vi "Micro-PL Drive Calibration v10.0.0.vi"() -> ()   [LabVIEW 2010]
uses:
  <vilib>/Utility/miscctls.llb/LVPointTypeDef.ctl
  subvi/ESA-C/TypeDefs/ESA-C Connection Settings.ctl
  <vilib>/Utility/file.llb/Write To Spreadsheet File (DBL).vi
panel:
  in  "GPIB-Port":u8=4 max=150 step=1
  in  "Start":bool
  out "Voltages":ext[][](array[numeric])
  out "Current Voltage":ext caption="Current (V)" format="%.1f"
  in  "Axis":u16(ring)=1 items=["X"=1, "Y"=2, "Z"=3]
  out "Progress":u8(slide) max=10 scale=0.0..100.0
  in  "Exit":bool
  in  "Voltage Step":dbl=1.0 caption="Step (V)" min=0.1 max=30.0 step=0.1
  # "Drive Calibration"
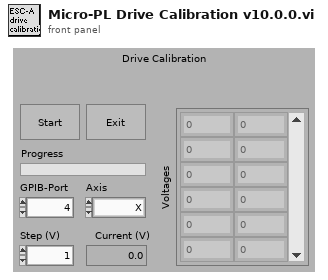
[diagram p1: front panel]
types:
  T1 = typedef "LVPointTypeDef.ctl" = cluster{"Horizontal":i16, "Vertical":i16}
  T2 = typedef "ESA-C Connection Settings.ctl" = cluster{"Objective GPIB-Port":i32, "Stage GPIB-Port":i32, "Drive Selector":u16, "Drive Velocity (V/s)":dbl}
  T3 = typedef "ESA-C Current Values.ctl" = cluster{"Voltages":cluster{"Drive X Voltage":dbl, "Drive Y Voltage":dbl, "Drive Z Voltage":dbl}, "Position":cluster{"Drive X Position":dbl, "Drive Y Position":dbl, "Drive Z Position":dbl}}
  T4 = cluster{"Drive X Voltage":dbl, "Drive Y Voltage":dbl, "Drive Z Voltage":dbl}
  T5 = enum32{"invalid app kind", "Development System", "Run Time System", "Student Edition", "Embedded LabVIEW", "Evaluation", "Custom"}
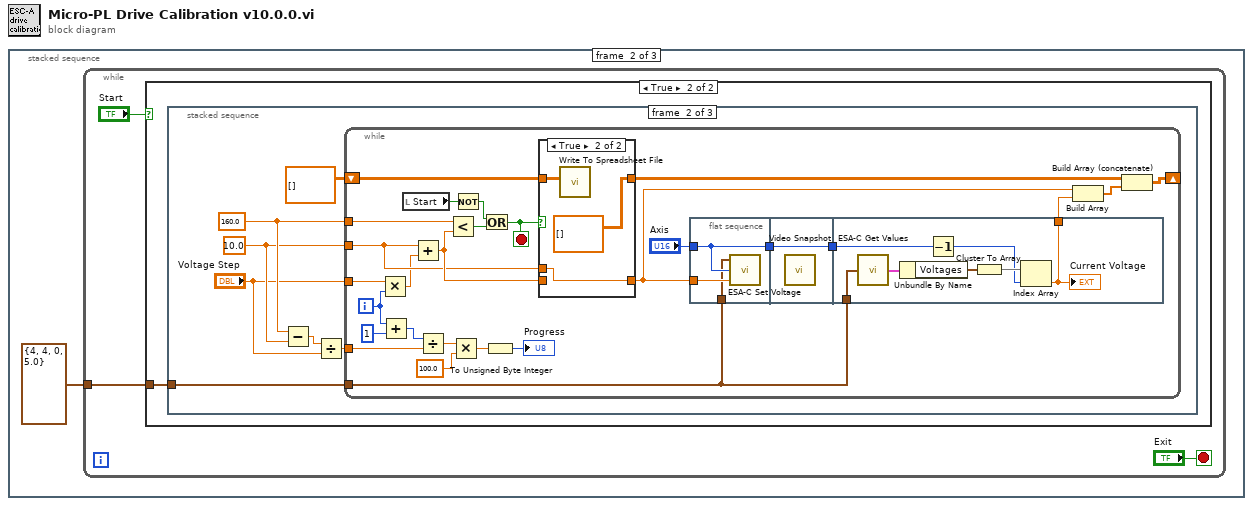
[diagram p0: block diagram]
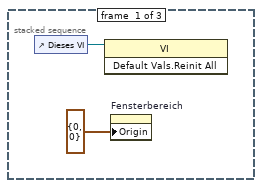
[diagram p2: hidden frame]
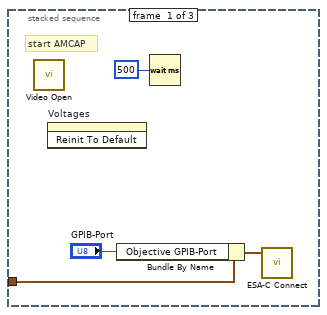
[diagram p4: hidden frame]
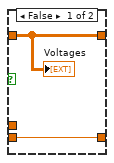
[diagram p5: hidden frame]
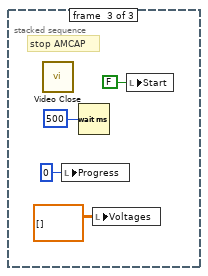
[diagram p6: hidden frame]
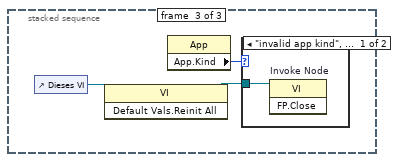
[diagram p7: hidden frame]
diagram:
  n1 = stacked-sequence {
    frame #0 {
      n2 = control-ref of="Dieses VI"() -> (w1:refnum<vi>)
      n3 = invoke class="VI" method="Default Vals.Reinit All"(reference=w1) -> ()  [unwired: 2 in, 3 out]
      n4 = property on="Fensterbereich" class="Pane"("Origin"=T1 {"Horizontal"=0, "Vertical"=0}) -> ()  [unwired: 2 in, 2 out]
    }
    frame #1 {
      n5 = while {
        tunnel: T2 {"Objective GPIB-Port"=4, "Stage GPIB-Port"=4, "Drive Selector"=0, "Drive Velocity (V/s)"=5.0} ("Drive Connection Settings") -> [w4]
        stop <- "Exit" stop-if-true
        n6 = case shown="True" "Start" {
          tunnel: w4 -> [_ w7]
          frame False {
          }
          frame True {
            n7 = stacked-sequence {
              tunnel: w7 -> [w10 w13 _]
              frame #0 {
                # "start AMCAP"
                n8 = call "Video Open.vi"() -> ()  [unwired: 11 in, 1 out]
                n9 = invoke on="Voltages" class="Arr (strikt)" method="Reinit To Default"() -> ()  [unwired: 3 in, 3 out]
                n10 = Bundle By Name(cluster=w10, "Objective GPIB-Port"="GPIB-Port") -> (w9:T2)
                n11 = Wait (ms)(milliseconds to wait=u32 500 ("Timer-Wert (ms)")) -> ()  [unwired: 1 out]
                n12 = call "ESA-C Connect.vi"("Drive Connection Settings"=w9) -> ()  [unwired: 3 in, 1 out]
              }
              frame #1 {
                w18 = 160.0 ("y")
                w17 = 10.0 ("y")
                n13 = Subtract(x=w18, y=w17) -> (x-y=w16:dbl)
                n14 = Divide(x=w16, y="Voltage Step") -> (x/y=w14:dbl)
                n15 = while {
                  tunnel: w17 -> [w32]
                  tunnel: "Voltage Step" -> [w21]
                  tunnel: w18 -> [w36]
                  tunnel: w14 -> [w38]
                  tunnel: w13 -> [w28]
                  shift-right: [w25] -> _
                  shift-left: dbl[][] [] -> [w24]
                  i -> [w22]
                  stop <- w43 stop-if-true
                  n16 = Multiply(x=w21, y=w22) -> (x*y=w20:dbl)
                  n17 = Add(x=w22, y=1) -> (x+y=w39:i32)
                  n18 = local read "Start"() -> (w34:bool)
                  n19 = Add(x=w32, y=w20) -> (x+y=w35:dbl)
                  n20 = Divide(x=w39, y=w38) -> (x/y=w44:dbl)
                  n21 = Less?(x=w36, y=w35) -> (x < y?=w45:bool)
                  n22 = Multiply(x=w44, y=100.0) -> (x*y=w42:dbl)
                  n23 = Not(x=w34) -> (.not. x?=w33:bool)
                  n24 = Or(x=w33, y=w45) -> (x .or. y?=w43:bool)
                  n25 = To Unsigned Byte Integer(number=w42) -> (unsigned 8bit integer=→"Progress":u8)
                  n26 = case shown="True" w43 {
                    tunnel: w35 -> [w58 _]
                    tunnel: w32 -> [_ w61]
                    tunnel: [w58 w61] -> w19
                    tunnel: w24 -> [w57 w60]
                    tunnel: [w57 dbl[][] []] -> w23
                    frame False {
                      "Voltages" <- w57
                    }
                    frame True {
                      n27 = call-poly <vilib>:"Write To Spreadsheet File.vi"("2D data"=w60) -> ()  [unwired: 7 in, 1 out]
                    }
                  }
                  n28 = flat-sequence {
                    tunnel: w19 -> [w47]
                    tunnel: "Axis" -> [w48]
                    tunnel: [w48] -> w31
                    tunnel: w28 -> [w46]
                    tunnel: [w49] -> w30
                    tunnel: w31 -> [w49]
                    tunnel: w30 -> [w51]
                    tunnel: w28 -> [w56]
                    tunnel: [w53] -> w27
                    frame #0 {
                      n29 = call "ESA-C Set Voltage.vi"("Voltage"=w47, "Axis"=w48, "Drive Connection Settings"=w46) -> ()  [unwired: 2 in]
                    }
                    frame #1 {
                      n30 = call "Video Snapshot.vi"() -> ()  [unwired: 11 in, 1 out]
                    }
                    frame #2 {
                      n31 = call "ESA-C Get Values.vi"("Drive Connection Settings"=w56) -> ("Drive Current Values"=w55:T3)
                      n32 = Unbundle By Name(w55) -> ("Voltages"=w54:T4)
                      n33 = Decrement(x=w51) -> (x-1=w50:u16)
                      n34 = Cluster To Array(cluster=w54) -> (array=w52:dbl[])
                      n35 = Index Array(array=w52, index=w50) -> (element=w53:dbl)
                      "Current Voltage" <- w53
                    }
                  }
                  n36 = Build Array(w19, w27) -> (w26:dbl[])
                  n37 = Build Array (concatenate)(w23, w26) -> (w25:dbl[][])
                }
              }
              frame #2 {
                # "stop AMCAP"
                n38 = call "Video Close.vi"() -> ()  [unwired: 11 in, 1 out]
                n39 = local write "Progress"(u8 0 ("Progress")) -> ()
                n40 = Wait (ms)(milliseconds to wait=u32 500 ("Timer-Wert (ms)")) -> ()  [unwired: 1 out]
                n41 = local write "Voltages"(ext[][] [] ("Voltages")) -> ()
                n42 = local write "Start"(FALSE ("Start")) -> ()
              }
            }
          }
        }
      }
    }
    frame #2 {
      n43 = control-ref of="Dieses VI"() -> (w68:refnum<vi>)
      n44 = invoke class="VI" method="Default Vals.Reinit All"(reference=w68) -> (reference out=w66:refnum<vi>)  [unwired: 2 in, 2 out]
      n45 = property class="App"() -> ("App.Kind"=w67:T5)  [unwired: 2 in, 2 out]
      n46 = case shown="\"invalid app kind\", Default" w67 {
        tunnel: w66 -> [w69 _]
        frame "invalid app kind", Default {
          n47 = invoke on="Invoke Node" class="VI" method="FP.Close"(reference=w69) -> ()  [unwired: 2 in, 3 out]
        }
        frame "Development System" {
        }
      }
    }
  }
